vi "路径.vi"() -> ()   [LabVIEW 2018]
panel:
  out "引用句柄输出":refnum<file>
  in  "文本 3":string
  out "添加的路径":path
  in  "文本 2":string
  in  "文本":string
  in  "文件（使用对话框）":path
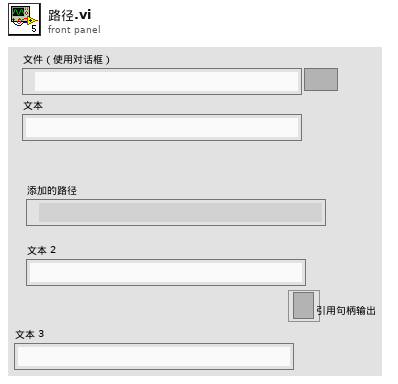
[diagram p1: front panel]
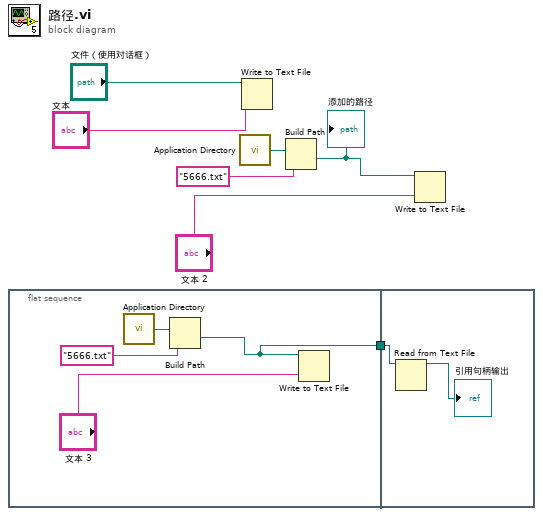
[diagram p0: block diagram]
diagram:
  n1 = flat-sequence {
    tunnel: [w8] -> w1
    tunnel: w1 -> [w13]
    frame #0 {
      n2 = call <vilib>:"Application Directory.vi"() -> ("Application Directory"=w10:path)
      n3 = Build Path(base path=w10, name or relative path="5666.txt" ("名称或相对路径")) -> (appended path=w8:path)
      n4 = Write to Text File(file (use dialog)=w8, text="文本 3") -> ()  [unwired: 2 in, 3 out]
    }
    frame #1 {
      n5 = Read from Text File(file (use dialog)=w13) -> (refnum out=→"引用句柄输出":refnum<file>)  [unwired: 3 in, 3 out]
    }
  }
  n6 = call <vilib>:"Application Directory.vi"() -> ("Application Directory"=w4:path)
  n7 = Write to Text File(file (use dialog)="文件（使用对话框）", text="文本") -> ()  [unwired: 2 in, 3 out]
  n8 = Build Path(base path=w4, name or relative path="5666.txt" ("名称或相对路径")) -> (appended path=w2:path)
  "添加的路径" <- w2
  n9 = Write to Text File(file (use dialog)=w2, text="文本 2") -> ()  [unwired: 2 in, 3 out]
